vi "extra_waitlines_read_flexRIO.vi"(11 "address extra waitlines IN":u32) -> (2 "extra waitline data":u32, 3 "address extra waitlines OUT":u32)   [LabVIEW 2010]
uses:
  <vilib>/rvi/DataTransferAndStorage/Container/XNode/niFpgaContainer.xnode
  <vilib>/rvi/Memory/Memory_Emulation/nirvimemoryEmulationManagerCache_GetValue.vi
  <vilib>/rvi/DataTransferAndStorage/Container/Common/niFpgaContainerGetUniqueNameForEmu.vi
  <vilib>/rvi/Memory/Memory_Emulation/nirvimemoryEmulationManagerCache_InsertValue.vi
  <vilib>/Utility/error.llb/Clear Errors.vi
  <vilib>/rvi/Memory/Memory_Emulation/nirvimemoryEmulationManagerCache_SetValue.vi
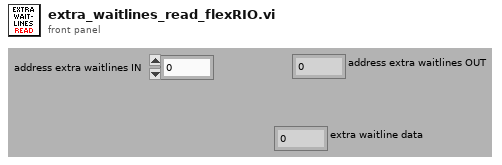
[diagram p1: front panel]
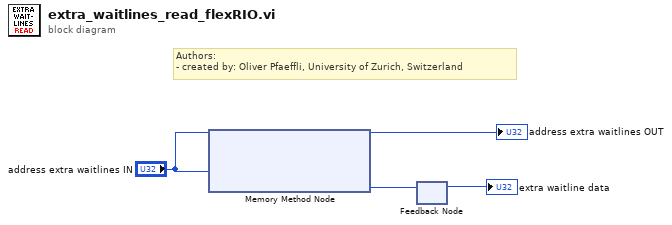
[diagram p0: block diagram]
diagram:
  # "Authors: \n- created by: Oliver Pfaeffli, University of Zurich, Switzerland"
  n1 = xnode ("Memory Method Node")("Address"="address extra waitlines IN") -> ("Data"=w2:u32)  [unwired: 1 in, 1 out]
  n2 = feedback #1() -> (→"extra waitline data":u32)  [unwired: 1 in]
  n3 = feedback-in #1(w2) -> ()
  "address extra waitlines OUT" <- "address extra waitlines IN"
